vi "getAllParagraphs.vi"(8 "error in (no error)":errorcluster, 11 "xwpfReader in":refnum<class "xwpfReader.lvclass">) -> (0 "error out":errorcluster, 1 "Paragraph Styles":refnum<class "Style.lvclass">[](array[class]), 2 "Paragraphs":string[](array[string]), 3 "xwpfReader out":refnum<class "xwpfReader.lvclass">)   [LabVIEW 2017, in "xwpfReader.lvclass"]
doc: "Get all the paragraphs."
uses:
  xwpfReader.lvclass
  Styles/Style/Style.lvclass
  xwpfReader.lvclass/xwpfReader.ctl
  C:/Users/Neo/Desktop/Dev_Tools_BR/LabVIEW_NPOI/lib/NPOI 2.1.1/NPOI.OOXML.dll
  lib/NPOI 2.1.1/NPOI.OOXML.dll
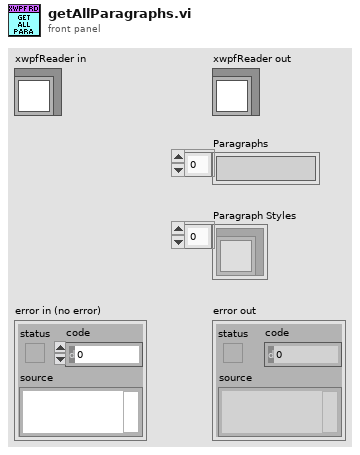
[diagram p1: front panel]
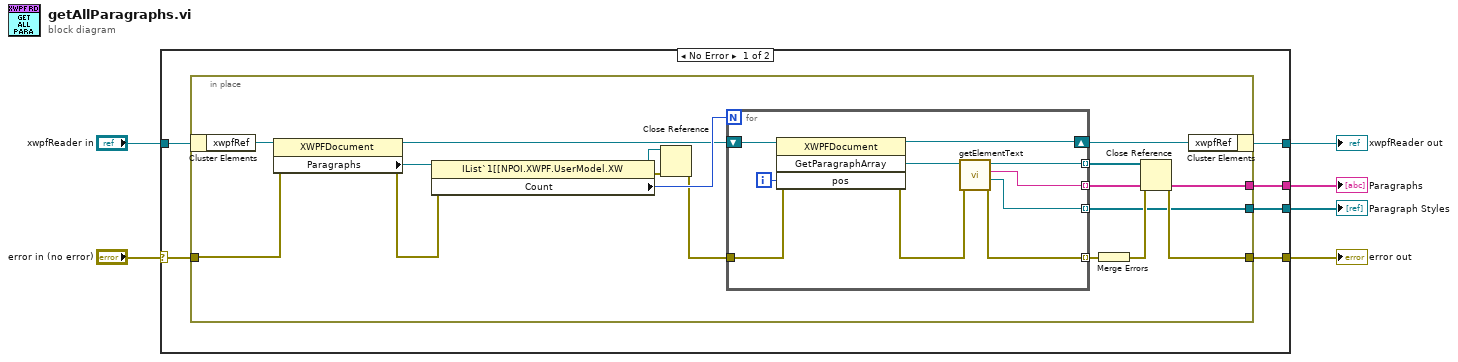
[diagram p0: block diagram]
diagram:
  n1 = case shown="No Error" "error in (no error)" {
    selector: "error in (no error)" -> [w10 w40]
    tunnel: [w9 w40] -> w5
    tunnel: [w12 w39] -> w3
    tunnel: "xwpfReader in" -> [w11 w39]
    tunnel: [w8 _] -> w2
    tunnel: [w7 _] -> w1
    frame No Error {
      n2 = in-place {
        in-place-border: w10 -> [w25]
        in-place-border: [w17] -> w9
        in-place-border: [w15] -> w8
        in-place-border: [w14] -> w7
        n3 = in-place-cluster #1(w11) -> ("xwpfRef"=w28:refnum<k24>)
        n4 = property class="XWPFDocument"(reference=w28, error in=w25) -> (reference out=w13:refnum<k24>, error out=w22:errorcluster, "Paragraphs"=w27:refnum<k24>)
        n5 = property class="IList`1[[NPOI.XWPF.UserModel.XW"(reference=w27, error in=w22) -> (reference out=w21:refnum<k24>, error out=w20:errorcluster, "Count"=w26:i32)
        n6 = Close Reference(reference=w21, error in (no error)=w20) -> (error out=w19:errorcluster)
        n7 = for {
          N: w26 -> [_]
          tunnel: [w32] -> w15 mode=indexing
          tunnel: [w33] -> w18 mode=indexing
          shift-right: [w37] -> w24
          shift-left: w13 -> [w35]
          tunnel: w19 -> [w36]
          tunnel: [w30] -> w23 mode=indexing
          tunnel: [w29] -> w14 mode=indexing
          i -> [w38]
          n8 = invoke class="XWPFDocument" method="GetParagraphArray"(reference=w35, error in=w36, "pos"=w38) -> (reference out=w37:refnum<k24>, error out=w31:errorcluster, "GetParagraphArray"=w34:refnum<k24>)  [unwired: 1 in, 1 out]
          n9 = call "getElementText.vi"("error in (no error)"=w31, "Paragraph in"=w34) -> ("error out"=w30:errorcluster, "Style"=w29:refnum<class "Style.lvclass">, "Text"=w32:string, "Paragraph out"=w33:refnum<k24>)  [unwired: 6 in]
        }
        n10 = Merge Errors(w23) -> (w16:errorcluster)
        n11 = Close Reference(reference=w18, error in (no error)=w16) -> (error out=w17:errorcluster)
        n12 = in-place-cluster #1("xwpfRef"=w24) -> (w12:refnum<class "xwpfReader.lvclass">)
      }
    }
    frame Error {
    }
  }
  "error out" <- w5
  "xwpfReader out" <- w3
  "Paragraphs" <- w2
  "Paragraph Styles" <- w1
